vi "Global Variables.vi"() -> ()   [LabVIEW 2018]
panel:
  out "TCP":bool
  in  "Version Format":string="%s %s FPGA: %d; RT: %d; MEM: 1\n%[^,;]; FW:\\s%d.%d.%d.%d.%s "
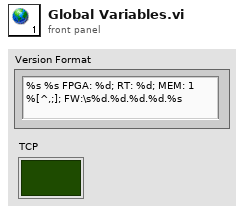
[diagram p1: front panel]
diagram:
